vi "manipulator Command Helper.vi"(7 "Description":string, 8 "Command Info In":T5, 11 "SubSystem Data":T1={"Operation"=enum."Reserve", "Immediate Parameters"={"Wrist Power"=0.0, "Cascade Power"=0.0}, "Griddy Parameters"={"Griddy Command"=enum."idle", "Flip Wrist?"=FALSE}, "Reset Parameters"={"Reset Wrist"=FALSE, "Reset Cascade"=FALSE}, "Shoot Cube Parameters"={"Shot Preset"=enum."shoot mid"}}) -> (0 "Command Info Out":T5, 1 "Command Timing":cluster{"Start Time (ms)":u32, "Iterations":i32}, 3 "SubSystem Data":T1={"Operation"=enum."Reserve", "Immediate Parameters"={"Wrist Power"=0.0, "Cascade Power"=0.0}, "Griddy Parameters"={"Griddy Command"=enum."idle", "Flip Wrist?"=FALSE}, "Reset Parameters"={"Reset Wrist"=FALSE, "Reset Cascade"=FALSE}, "Shoot Cube Parameters"={"Shot Preset"=enum."shoot mid"}})   [LabVIEW 2020]
doc: "This VI shouldn't not be used directly, but is the core functionality of any given command. It is the primary communication path to the controller and stores the current command info."
uses:
  manipulator Setpoints.ctl
  manipulator Operations.ctl
  Typedefs/Teleop Manipulator Commands.ctl
  Typedefs/Cube Shooting Presets.ctl
  <vilib>/Rock Robotics/WPI/Framework/Command Status Info.ctl
  <vilib>/Rock Robotics/WPI/Framework/Completion Status.ctl
  <vilib>/Rock Robotics/WPI/Framework/Completion Notifier.ctl
  manipulator Published Globals.vi
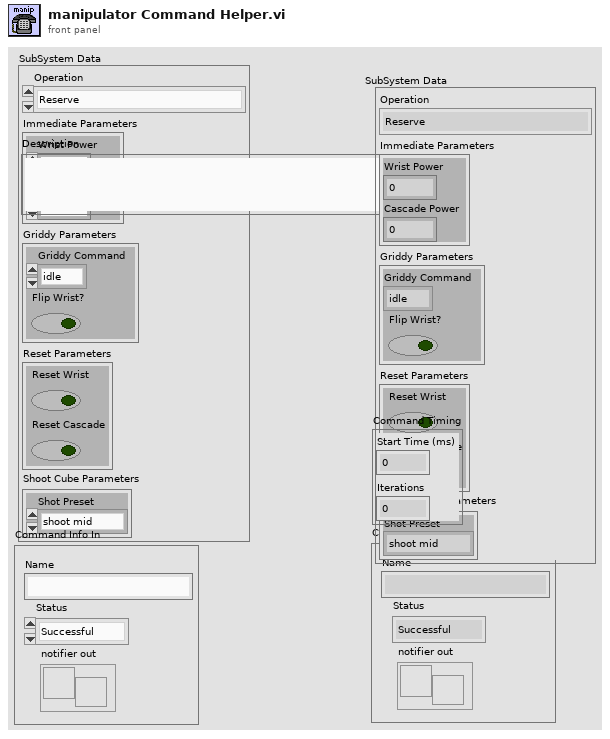
[diagram p1: front panel]
types:
  T1 = typedef "manipulator Setpoints.ctl" = cluster{"Operation":T2, "Immediate Parameters":cluster{"Wrist Power":dbl, "Cascade Power":dbl}, "Griddy Parameters":cluster{"Griddy Command":T3, "Flip Wrist?":bool}, "Reset Parameters":cluster{"Reset Wrist":bool, "Reset Cascade":bool}, "Shoot Cube Parameters":cluster{"Shot Preset":T4}}
  T2 = typedef "manipulator Operations.ctl" = enum16{"Reserve", "Read Current", "Immediate", "Reset Manipulator", "Grid-dy", "Shoot Cubes"}
  T3 = typedef "Teleop Manipulator Commands.ctl" = enum16{"idle", "intake cone sideways", "intake cone upright", "intake cone feeder", "intake cube feeder", "intake cube", "score low cone", "score low cube", "score mid cone", "score mid cube", "score high cone", "score high cube", "score mid cone up"}
  T4 = typedef "Cube Shooting Presets.ctl" = enum16{"shoot low", "shoot mid", "shoot high"}
  T5 = typedef "Command Status Info.ctl" = cluster{"Name":string, "Status":T6, "notifier out":T7}
  T6 = typedef "Completion Status.ctl" = enum16{"Successful", "Aborted", "Incomplete"}
  T7 = typedef "Completion Notifier.ctl" = refnum<notifier>
  T8 = cluster{"Current Command":T1, "Command Timing":cluster{"Start Time (ms)":u32, "Iterations":i32}, "Command Arguments":cluster{"Command Info":T5, "Description":string, "Default Command":T1, "queue out":refnum<queue>, "Subsystem Name":string}}
  T9 = cluster{"SubSystem Data":T1, "Command Info In":T5, string}
  T10 = cluster{"Command Info":T5, "Description":string, "Default Command":T1, "queue out":refnum<queue>, "Subsystem Name":string}
  T11 = cluster{"SubSystem Data":T1, "Command Info In":T5, "Description":string}
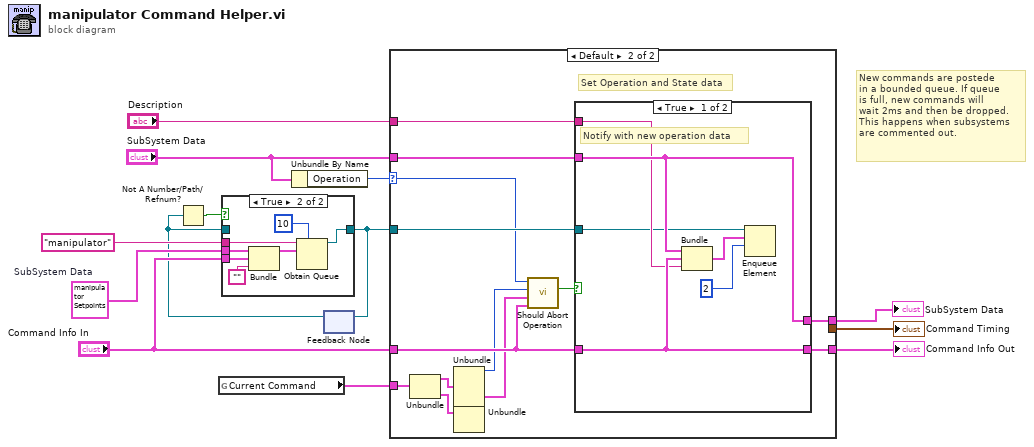
[diagram p0: block diagram]
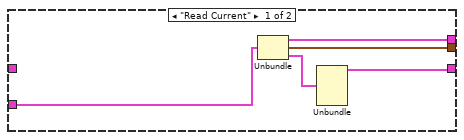
[diagram p3: hidden frame]
diagram:
  w7 = T1 {"Operation"=enum."Reserve", "Immediate Parameters"={"Wrist Power"=0.0, "Cascade Power"=0.0}, "Griddy Parameters"={"Griddy Command"=enum."idle", "Flip Wrist?"=FALSE}, "Reset Parameters"={"Reset Wrist"=FALSE, "Reset Cascade"=FALSE}, "Shoot Cube Parameters"={"Shot Preset"=enum."shoot mid"}}  # SubSystem Data
  # "New commands are postede\nin a bounded queue. If queue\nis full, new commands will\nwait 2ms and then be dropped.\nThis happens when subsystems\nare commented out."
  n1 = global read "manipulator Published Globals.vi" "Current Command"() -> (w1:T8)
  n2 = Unbundle By Name("SubSystem Data") -> ("Operation"=w12:T2)
  n3 = feedback #1() -> (w4:refnum<queue>)  [unwired: 1 in]
  n4 = Not A Number/Path/Refnum?(number/path/refnum=w4) -> (NaN/Path/Refnum?=w5:bool)
  n5 = case shown="True" w5 {
    tunnel: "manipulator" -> [_ w18]
    tunnel: [w14 w16] -> w10
    tunnel: w7 -> [_ w21]
    tunnel: "Command Info In" -> [_ w20]
    tunnel: w4 -> [w14 _]
    frame False {
    }
    frame True {
      n6 = Bundle("SubSystem Data"=w21, "Command Info In"=w20, "") -> (w17:T9)  [unwired: 1 in]
      n7 = Obtain Queue(max queue size (-1, unlimited)=10, name (unnamed)=w18, element data type=w17) -> (queue out=w16:refnum<queue>)  [unwired: 2 in, 2 out]
    }
  }
  n8 = feedback-in #1(w10) -> ()
  n9 = case shown="Default" w12 {
    selector: w12 -> [_ w34]
    tunnel: [w25 w36] -> w6
    tunnel: w10 -> [_ w38]
    tunnel: "SubSystem Data" -> [_ w39]
    tunnel: [w24 w37] -> w9
    tunnel: "Command Info In" -> [_ w33]
    tunnel: "Description" -> [_ w32]
    tunnel: [w23 _] -> w2
    tunnel: w1 -> [w22 w31]
    frame "Read Current" {
      n10 = Unbundle(w22) -> ("Current Command"=w25:T1, "Command Timing"=w23:cluster{"Start Time (ms)":u32, "Iterations":i32}, "Command Arguments"=w26:T10)
      n11 = Unbundle(w26) -> ("Command Info"=w24:T5)  [unwired: 4 out]
    }
    frame Default {
      # "Set Operation and State data"
      n12 = Unbundle(w31) -> ("Current Command"=w30:T1, "Command Arguments"=w28:T10)  [unwired: 1 out]
      n13 = Unbundle(w30) -> ("Operation"=w29:T2)  [unwired: 4 out]
      n14 = Unbundle(w28) -> ("Command Info"=w27:T5)  [unwired: 4 out]
      n15 = call <vilib>:"Should Abort Operation.vi"("New Command Info"=w33, "Command Info"=w27, "Current Operation"=w29, "New Operation"=w34) -> ("Execute"=w35:bool)  [unwired: 7 in]
      n16 = case shown="True" w35 {
        tunnel: [w45 _] -> w36
        tunnel: w39 -> [w45 _]
        tunnel: w38 -> [w42 _]
        tunnel: [w44 w46] -> w37
        tunnel: w33 -> [w44 w46]
        tunnel: w32 -> [w43 _]
        frame True {
          # "Notify with new operation data"
          n17 = Bundle("SubSystem Data"=w45, "Command Info In"=w44, "Description"=w43) -> (w41:T11)  [unwired: 1 in]
          n18 = Enqueue Element(queue=w42, element=w41, timeout in ms (-1)=2 ("max queue size (-1, unlimited)")) -> ()  [unwired: 1 in, 3 out]
        }
        frame False {
          # "This operation will not be\nexecuted. Upstream command\nwas aborted."
        }
      }
    }
  }
  "Command Info Out" <- w9
  "SubSystem Data" <- w6
  "Command Timing" <- w2
